vi "WebView.JSONEditor_Init.vi"(8 "Error In":errorcluster, 10 "WebView2 Control in":refnum<k24>(container), 11 "Object in":refnum<class "WebView.JSONEditor.lvclass">) -> (0 "Error Out":errorcluster, 3 "object out":refnum<class "WebView.JSONEditor.lvclass">)   [LabVIEW 2024, in "WebView.JSONEditor.lvclass"]
uses:
  WebView.JSONEditor.lvclass
  C:/Git/WebView-Components/WebView_class/WebView.lvclass
  Event Handler.vi
  WebView.JSONEditor.lvclass/WebView.JSONEditor.ctl
  WebView_class/WebView.lvclass
  C:/Git/WebView-Components/WebView.JSONEditor_class/WebView.JSONEditor.lvclass
  <vilib>/IlluminatedG/IG ExecAnchor/ExecAnchor/ExecAnchor.lvclass
  <vilib>/sklein/WebView2/Libs/Microsoft.Web.WebView2.WinForms.dll
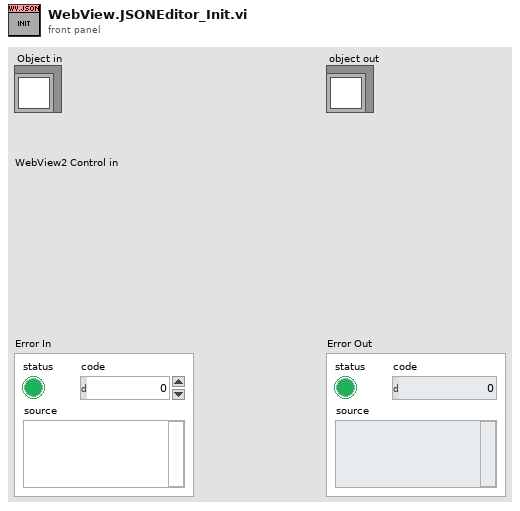
[diagram p1: front panel]
types:
  T1 = typedef "WebView.lvclass/Events--cluster.ctl" = cluster{"Navigation Complete Event":refnum<user-event>, "Source Changed Event":refnum<user-event>, "Document Title Changed Event":refnum<user-event>, "Status Bar Text Changed":refnum<user-event>, "Web Message Received":refnum<user-event>, "Window Close Requested":refnum<user-event>, "DOM Loaded":refnum<user-event>, "Navigation Started Event":refnum<user-event>}
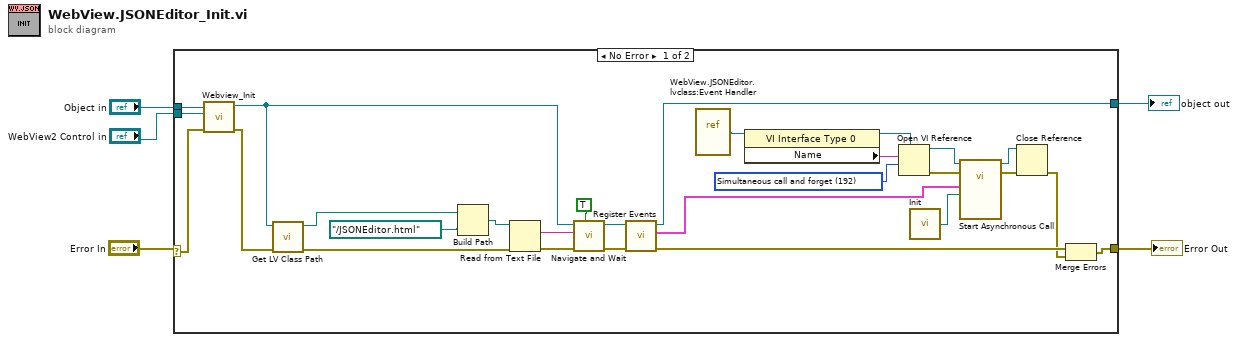
[diagram p0: block diagram]
diagram:
  n1 = case shown="No Error" "Error In" {
    selector: "Error In" -> [w33 w34]
    tunnel: [w30 w35] -> w5
    tunnel: "Object in" -> [w32 w35]
    tunnel: [w7 w34] -> w2
    tunnel: "WebView2 Control in" -> [w20 _]
    frame No Error {
      w12 = 192 items=["Record modifications"=1, "Open templates for editing"=2, "Prompt user to save"=4, "Prepare for reentrant run"=8, "Prompt to find missing subVIs"=16, "Hide loading dialog box"=32, "Enable simultaneous calls"=64, "Prepare to call and forget"=128, "Simultaneous call and forget"=192, "Prepare to call and collect"=256, "Simultaneous call and collect"=320]
      n2 = call "Webview_Init.vi"("Error In"=w33, "WebView2 Control in"=w20, "object in"=w32) -> ("Error Out"=w26:errorcluster, "object out"=w27:refnum<class "WebView.JSONEditor.lvclass">)  [unwired: 7 in]
      n3 = call <vilib>:"Get LV Class Path.vi"("error in (no error)"=w26, "object"=w27) -> ("error out"=w25:errorcluster, "class path"=w24:path)  [unwired: 8 in]
      n4 = Build Path(base path=w24, name or relative path=path "../JSONEditor.html") -> (appended path=w22:path)
      n5 = Read from Text File(file (use dialog)=w22, error in=w25) -> (text=w28:string, error out=w29:errorcluster)  [unwired: 2 in, 2 out]
      n6 = call "Navigate and Wait.vi"("html Source (URL)"=TRUE, "Error In"=w29, "Source"=w28, "object in"=w27) -> ("Error Out"=w21:errorcluster, "object out"=w31:refnum<class "WebView.JSONEditor.lvclass">)  [unwired: 5 in, 1 out]
      n7 = call-dynamic "Register Events.vi"("Error In"=w21, "object in"=w31) -> ("Error Out"=w8:errorcluster, "Events"=w11:T1, "object out"=w30:refnum<class "WebView.JSONEditor.lvclass">)  [unwired: 7 in]
      n8 = vi-ref "WebView.JSONEditor.lvclass:Event Handler.vi"() -> (w18:refnum<vi>)
      n9 = property class="VI Interface Type 0"(reference=w18) -> (reference out=w16:refnum<vi>, "Name"=w17:string)  [unwired: 1 in, 1 out]
      n10 = Open VI Reference(type specifier VI Refnum (for type only)=w16, vi path=w17, options=w12) -> (vi reference=w19:refnum<vi>, error out=w15:errorcluster)  [unwired: 3 in]
      n11 = call <vilib>:"Init.vi"() -> ("ExecAnchor out"=w10:refnum<class "ExecAnchor.lvclass">)  [unwired: 7 in]
      n12 = call-by-ref "Start Asynchronous Call"(reference=w19, error in=w15, "ExecAnchor in"=w10, "Events"=w11) -> (reference out=w13:refnum<vi>, error out=w14:errorcluster)  [unwired: 9 in, 1 out]
      n13 = Close Reference(reference=w13, error in (no error)=w14) -> (error out=w6:errorcluster)
      n14 = Merge Errors(w8, w6) -> (w7:errorcluster)
    }
    frame Error {
    }
  }
  "object out" <- w5
  "Error Out" <- w2
